vi "CélulaDessalinizadora.vi"() -> ()   [LabVIEW 2014]
panel:
  in  "NÚMERO DE CICLOS":dbl
  in  "Liga/Desliga":bool
  in  "Escolha: Porta Serial":refnum<visa-resource-name>="COM3"
  out "Dessorção":bool
  out "Adssorção":bool
  out "Single-Pass":bool
  out "Batch":bool
  in  "BATCH / SINGLE PASS":bool
  out "CORRENTE (A)":dbl(graph)
  out "pH":dbl(graph)
  out "CONDUTIVIDADE (us/cm)":dbl(graph)
  in  "?":enum32{"POTENCIOSTÁTICO", "GALVANOSTÁTICO"}(tab)
  in  "CONDUTIVIDADE \nMÁXIMA NA DESSORÇÃO P":dbl
  in  "TEMPO DE DESSOR敲O P":dbl
  in  "CONDUTIVIDADE \nMÍNIMA NA ADSORÇÃO P":dbl
  in  "TEMPO DE ADSOR敲O P":dbl
  in  "POTENCIAL DE CORTE\nNA DESSOR敲O (V) G":dbl
  in  "POTENCIAL DE CORTE\nNA ADSOR敲O (V) G":dbl
  in  "CONDUTIVIDADE \nMÁXIMA NA DESSORÇÃO G":dbl
  in  "TEMPO DE DESSOR敲O G":dbl
  in  "CONDUTIVIDADE \nMÍNIMA NA ADSORÇÃO G":dbl
  in  "TEMPO DE ADSOR敲O G":dbl
  # "s"
  # "s"
  # "us/cm"
  # "s"
  # "us/cm"
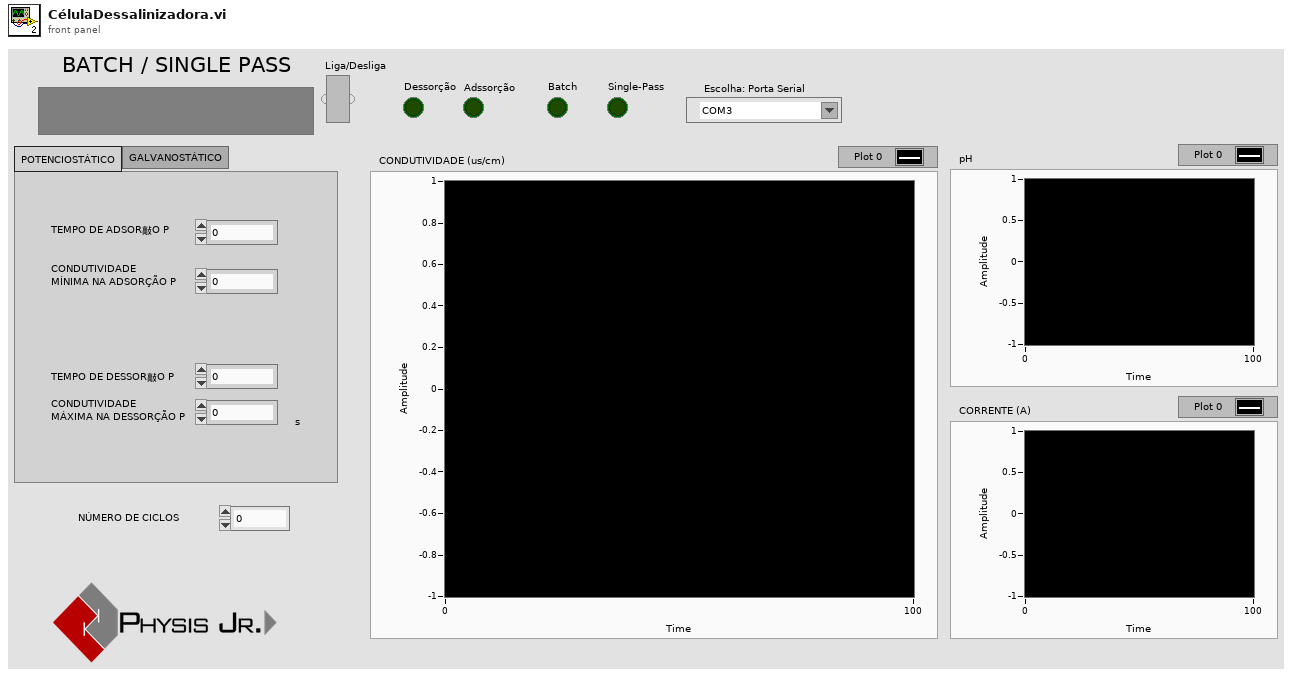
[diagram p1: front panel]
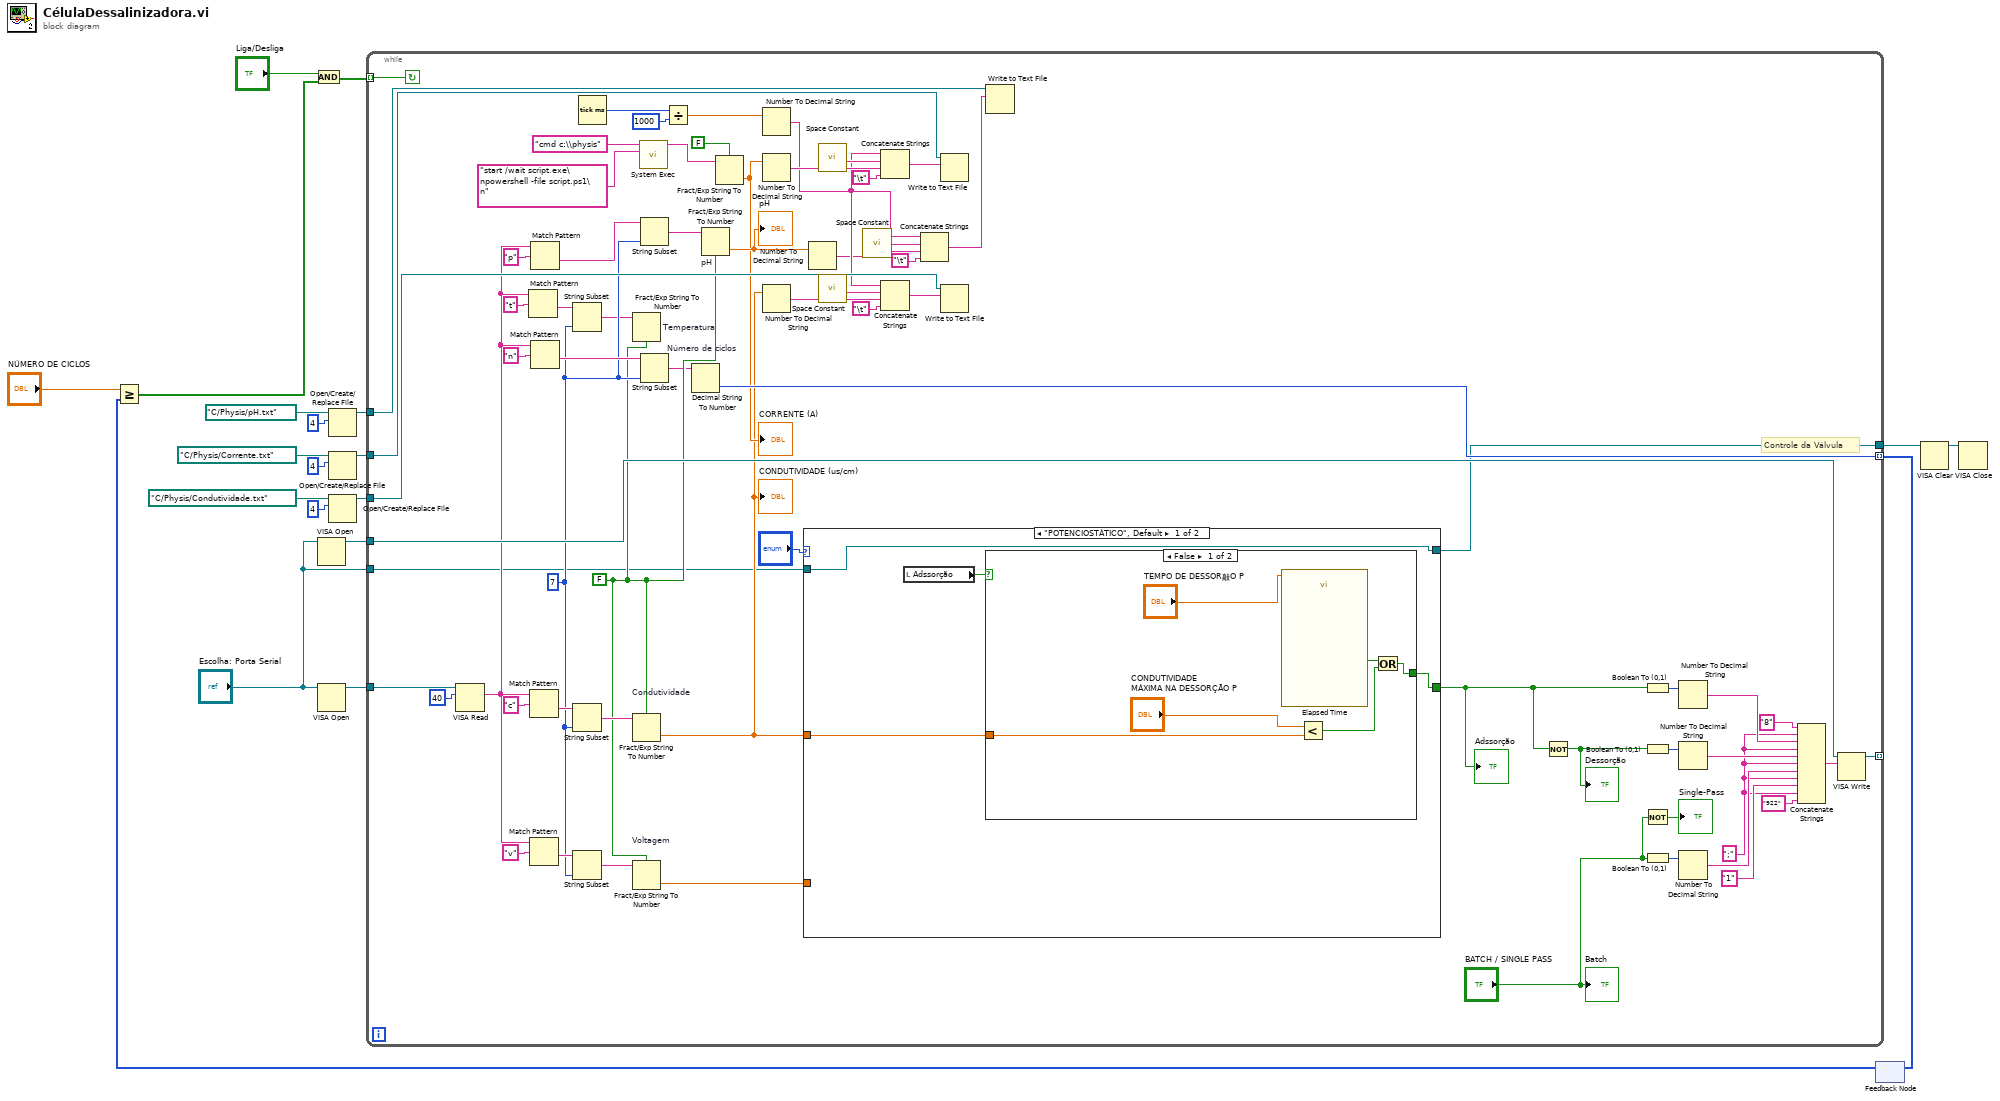
[diagram p0: block diagram]
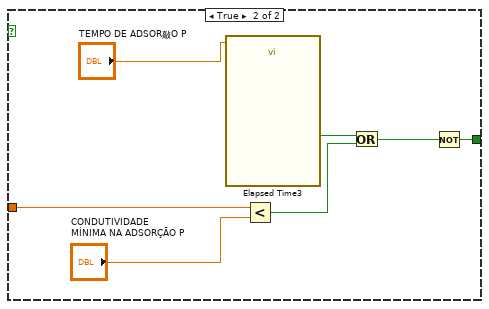
[diagram p2: hidden frame]
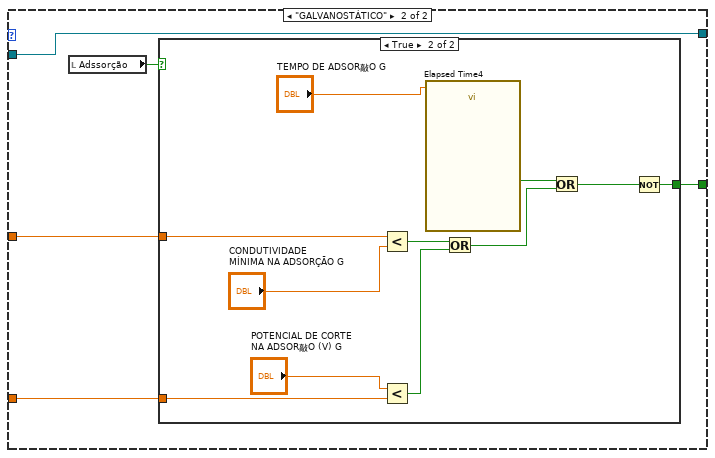
[diagram p3: hidden frame]
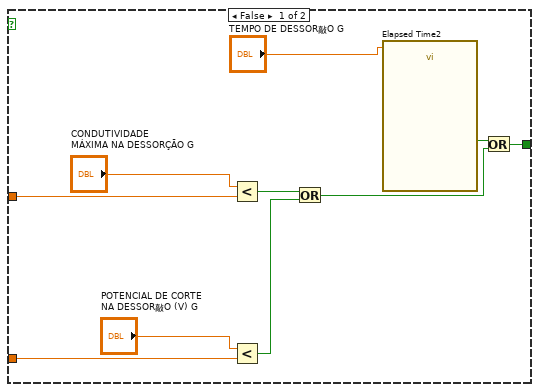
[diagram p4: hidden frame]
diagram:
  n1 = VISA Open(VISA resource name="Escolha: Porta Serial") -> (VISA resource name=w13:refnum<visa-resource-name>)  [unwired: 4 in, 1 out]
  n2 = VISA Open(VISA resource name="Escolha: Porta Serial") -> (VISA resource name=w14:refnum<visa-resource-name>)  [unwired: 4 in, 1 out]
  n3 = Open/Create/Replace File(file path (use dialog)=path "C:/Physis/pH.txt", operation (0:open)=4) -> (refnum out=w17:refnum<file>)  [unwired: 4 in, 2 out]
  n4 = Open/Create/Replace File(file path (use dialog)=path "C:/Physis/Corrente.txt", operation (0:open)=4) -> (refnum out=w16:refnum<file>)  [unwired: 4 in, 2 out]
  n5 = Open/Create/Replace File(file path (use dialog)=path "C:/Physis/Condutividade.txt", operation (0:open)=4) -> (refnum out=w19:refnum<file>)  [unwired: 4 in, 2 out]
  n6 = feedback #1() -> (w10:i32[])  [unwired: 1 in]
  n7 = Greater Or Equal?(x="NÚMERO DE CICLOS", y=w10) -> (x >= y?=w5:bool[])
  n8 = And(x="Liga/Desliga", y=w5) -> (x .and. y?=w4:bool[])
  n9 = while {
    tunnel: w19 -> [w89]
    tunnel: w17 -> [w88]
    tunnel: w16 -> [w87]
    tunnel: w14 -> [w74]
    tunnel: w13 -> [w73]
    tunnel: [w72] -> _ mode=indexing
    tunnel: w4 -> [w71] mode=indexing
    tunnel: [w70] -> w11 mode=indexing
    tunnel: "Escolha: Porta Serial" -> [w27]
    tunnel: [w26] -> w1
    stop <- w71 continue-if-true
    w40 = FALSE
    w46 = 7
    w77 = ";"
    # "Controle da Válvula"
    n10 = VISA Read(VISA resource name=w74, byte count=40) -> (read buffer=w52:string)  [unwired: 1 in, 3 out]
    n11 = Match Pattern(string=w52, regular expression="t") -> (after substring=w50:string)  [unwired: 1 in, 3 out]
    n12 = Match Pattern(string=w52, regular expression="c") -> (after substring=w49:string)  [unwired: 1 in, 3 out]
    n13 = Match Pattern(string=w52, regular expression="v") -> (after substring=w48:string)  [unwired: 1 in, 3 out]
    n14 = Match Pattern(string=w52, regular expression="p") -> (after substring=w51:string)  [unwired: 1 in, 3 out]
    n15 = Match Pattern(string=w52, regular expression="n") -> (after substring=w47:string)  [unwired: 1 in, 3 out]
    n16 = String Subset(string=w50, length (rest)=w46) -> (substring=w44:string)  [unwired: 1 in]
    n17 = String Subset(string=w49, length (rest)=w46) -> (substring=w43:string)  [unwired: 1 in]
    n18 = String Subset(string=w48, length (rest)=w46) -> (substring=w42:string)  [unwired: 1 in]
    n19 = Tick Count (ms)() -> (millisecond timer value=w39:u32)
    n20 = Fract/Exp String To Number "Temperatura"(use system decimal point (T)=w40, string=w44) -> ()  [unwired: 2 in, 2 out]
    n21 = Fract/Exp String To Number "Condutividade"(use system decimal point (T)=w40, string=w43) -> (number=w29:dbl)  [unwired: 2 in, 1 out]
    "CONDUTIVIDADE (us/cm)" <- w29
    n22 = Fract/Exp String To Number "Voltagem"(use system decimal point (T)=w40, string=w42) -> (number=w28:dbl)  [unwired: 2 in, 1 out]
    n23 = call <vilib>:"System Exec.vi"("standard input"="start /wait script.exe\npowershell -file script.ps1\n", "command line"="cmd c:\\physis") -> ("standard output"=w33:string)  [unwired: 6 in, 3 out]
    n24 = String Subset(string=w51, length (rest)=w46) -> (substring=w45:string)  [unwired: 1 in]
    n25 = String Subset(string=w47, length (rest)=w46) -> (substring=w36:string)  [unwired: 1 in]
    n26 = Divide(x=w39, y=1000) -> (x/y=w37:dbl)
    n27 = Decimal String To Number "Número de ciclos"(string=w36) -> (number=w70:i32)  [unwired: 2 in, 1 out]
    n28 = Fract/Exp String To Number "pH"(use system decimal point (T)=w40, string=w45) -> (number=w41:dbl)  [unwired: 2 in, 1 out]
    "pH" <- w41
    n29 = Fract/Exp String To Number(use system decimal point (T)=FALSE, string=w33) -> (number=w32:dbl)  [unwired: 2 in, 1 out]
    "CORRENTE (A)" <- w32
    n30 = Number To Decimal String(number=w37) -> (decimal integer string=w60:string)  [unwired: 1 in]
    n31 = Number To Decimal String(number=w32) -> (decimal integer string=w61:string)  [unwired: 1 in]
    n32 = Number To Decimal String(number=w29) -> (decimal integer string=w67:string)  [unwired: 1 in]
    n33 = case shown="\"POTENCIOSTÁTICO\", Default" "?" {
      tunnel: [w92 w110] -> w69
      tunnel: w29 -> [w91 w109]
      tunnel: w28 -> [_ w108]
      tunnel: w27 -> [w90 w107]
      tunnel: [w90 w107] -> w26
      frame "POTENCIOSTÁTICO", Default {
        n34 = local read "Adssorção"() -> (w93:bool)
        n35 = case shown="False" w93 {
          tunnel: [w98 w106] -> w92
          tunnel: w91 -> [w96 w102]
          frame False {
            n36 = call "Elapsed Time"("Time Target (s)"="TEMPO DE DESSOR敲O P") -> ("Time has Elapsed"=w94:bool)  [unwired: 11 in, 7 out]
            n37 = Less?(x="CONDUTIVIDADE \nMÁXIMA NA DESSORÇÃO P", y=w96) -> (x < y?=w97:bool)
            n38 = Or(x=w94, y=w97) -> (x .or. y?=w98:bool)
          }
          frame True {
            n39 = call "Elapsed Time3"("Time Target (s)"="TEMPO DE ADSOR敲O P") -> ("Time has Elapsed"=w103:bool)  [unwired: 11 in, 7 out]
            n40 = Less?(x=w102, y="CONDUTIVIDADE \nMÍNIMA NA ADSORÇÃO P") -> (x < y?=w100:bool)
            n41 = Or(x=w103, y=w100) -> (x .or. y?=w105:bool)
            n42 = Not(x=w105) -> (.not. x?=w106:bool)
          }
        }
      }
      frame "GALVANOSTÁTICO" {
        n43 = local read "Adssorção"() -> (w111:bool)
        n44 = case shown="True" w111 {
          tunnel: [w120 w131] -> w110
          tunnel: w109 -> [w112 w122]
          tunnel: w108 -> [w114 w124]
          frame False {
            n45 = Less?(x="CONDUTIVIDADE \nMÁXIMA NA DESSORÇÃO G", y=w112) -> (x < y?=w117:bool)
            n46 = Less?(x="POTENCIAL DE CORTE\nNA DESSOR敲O (V) G", y=w114) -> (x < y?=w118:bool)
            n47 = Or(x=w117, y=w118) -> (x .or. y?=w119:bool)
            n48 = call "Elapsed Time2"("Time Target (s)"="TEMPO DE DESSOR敲O G") -> ("Time has Elapsed"=w115:bool)  [unwired: 11 in, 7 out]
            n49 = Or(x=w115, y=w119) -> (x .or. y?=w120:bool)
          }
          frame True {
            n50 = Less?(x=w122, y="CONDUTIVIDADE \nMÍNIMA NA ADSORÇÃO G") -> (x < y?=w129:bool)
            n51 = Less?(x="POTENCIAL DE CORTE\nNA ADSOR敲O (V) G", y=w124) -> (x < y?=w127:bool)
            n52 = call "Elapsed Time4"("Time Target (s)"="TEMPO DE ADSOR敲O G") -> ("Time has Elapsed"=w125:bool)  [unwired: 11 in, 7 out]
            n53 = Or(x=w129, y=w127) -> (x .or. y?=w128:bool)
            n54 = Or(x=w125, y=w128) -> (x .or. y?=w132:bool)
            n55 = Not(x=w132) -> (.not. x?=w131:bool)
          }
        }
      }
    }
    "Adssorção" <- w69
    n56 = Number To Decimal String(number=w41) -> (decimal integer string=w59:string)  [unwired: 1 in]
    n57 = call <vilib>:"Space Constant.vi"() -> ("String"=w64:string)
    n58 = call <vilib>:"Space Constant.vi"() -> ("String"=w68:string)
    n59 = call <vilib>:"Space Constant.vi"() -> ("String"=w63:string)
    n60 = Concatenate Strings(w60, w64, w61, "\t") -> (w65:string)
    n61 = Concatenate Strings(w60, w68, w67, "\t") -> (w66:string)
    n62 = Concatenate Strings(w60, w63, w59, "\t") -> (w62:string)
    n63 = Write to Text File(file (use dialog)=w87, text=w65) -> ()  [unwired: 2 in, 3 out]
    n64 = Write to Text File(file (use dialog)=w89, text=w66) -> ()  [unwired: 2 in, 3 out]
    n65 = Write to Text File(file (use dialog)=w88, text=w62) -> ()  [unwired: 2 in, 3 out]
    n66 = Not(x=w69) -> (.not. x?=w86:bool)
    "Dessorção" <- w86
    n67 = Boolean To (0,1)(Boolean=w69) -> (0, 1=w83:i16)
    n68 = Boolean To (0,1)(Boolean=w86) -> (0, 1=w82:i16)
    n69 = Not(x="BATCH / SINGLE PASS") -> (.not. x?=→"Single-Pass":bool)
    n70 = Boolean To (0,1)(Boolean="BATCH / SINGLE PASS") -> (0, 1=w84:i16)
    n71 = Number To Decimal String(number=w83) -> (decimal integer string=w81:string)  [unwired: 1 in]
    n72 = Number To Decimal String(number=w82) -> (decimal integer string=w80:string)  [unwired: 1 in]
    n73 = Number To Decimal String(number=w84) -> (decimal integer string=w79:string)  [unwired: 1 in]
    n74 = Concatenate Strings("8", w77, w81, w77, w80, w77, w79, w77, "1", w77, "922") -> (w75:string)
    n75 = VISA Write(VISA resource name=w73, write buffer=w75) -> (VISA resource name out=w72:refnum<visa-resource-name>)  [unwired: 1 in, 2 out]
    "Batch" <- "BATCH / SINGLE PASS"
  }
  n76 = feedback-in #1(w11) -> ()
  n77 = VISA Clear(VISA resource name=w1) -> (VISA resource name out=w3:refnum<visa-resource-name>)  [unwired: 1 in, 1 out]
  n78 = VISA Close(VISA resource name=w3) -> ()  [unwired: 1 in, 1 out]
